vi "OPC Query.vi"(8 "error in (no error)":errorcluster, 11 "VISA resource name":refnum<visa-resource-name>) -> (0 "error out":errorcluster, 2 "*OPC? Returns":i16, 3 "VISA resource name out":refnum<visa-resource-name>)   [LabVIEW 2017, in "ADCMT7351_ADC.lvlib"]
doc: "This VI waits for operation by the instruments to be completed, using *OPC? command."
uses:
  ADCMT7351_ADC.lvlib
  Instance           1 17Saved   OPC Query .vi
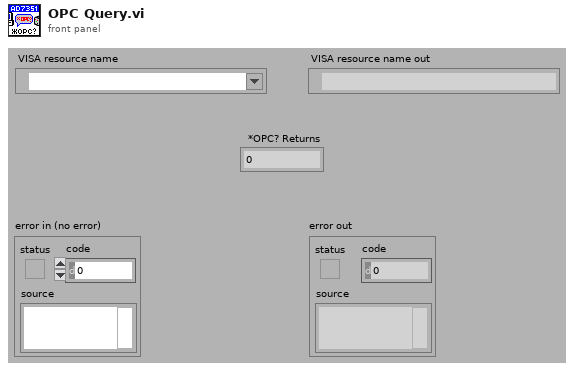
[diagram p1: front panel]
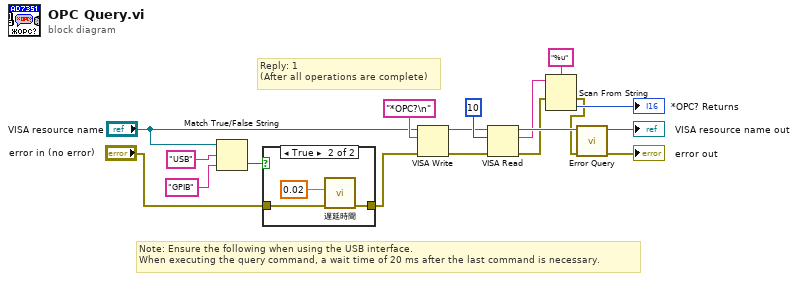
[diagram p0: block diagram]
diagram:
  # "Reply: 1\n(After all operations are complete)"
  # "Note: Ensure the following when using the USB interface.\nWhen executing the query command, a wait time of 20 ms after the last command is necessary."
  n1 = Match True/False String(2:"GPIB" ("false文字列"), 3:"USB" ("true文字列"), 4:"VISA resource name") -> (0:w5:bool)  [unwired: 1 out]
  n2 = case shown="True" w5 {
    tunnel: [w19 w21] -> w7
    tunnel: "error in (no error)" -> [w19 w20]
    frame False {
    }
    frame True {
      n3 = call "遅延時間"("error in (no error)"=w20, "Delay Time (s)"=0.02) -> ("error out"=w21:errorcluster)  [unwired: 9 in]
    }
  }
  n4 = VISA Write(VISA resource name="VISA resource name", write buffer="*OPC?\n" ("*OPC? Command"), error in (no error)=w7) -> (VISA resource name out=w4:refnum<visa-resource-name>, error out=w3:errorcluster)  [unwired: 1 out]
  n5 = VISA Read(VISA resource name=w4, byte count=u32 10 ("Bytes to Read"), error in (no error)=w3) -> (VISA resource name out=w16:refnum<visa-resource-name>, read buffer=w11:string, error out=w2:errorcluster)  [unwired: 1 out]
  n6 = Scan From String(format string="%u" ("Format String"), input string=w11, error in=w2) -> (error out=w1:errorcluster, output 1=→"*OPC? Returns":i16)  [unwired: 2 in, 2 out]
  n7 = call "Error Query.vi"("error in (no error)"=w1, "VISA resource name"=w16) -> ("error out"=→"error out":errorcluster, "VISA resource name out"=→"VISA resource name out":refnum<visa-resource-name>)  [unwired: 6 in, 2 out]
